vi "calibrateEvent.vi"(8 "error in (no error)":errorcluster, 11 "RampEvent in":refnum<class "RampEvent.lvclass">) -> (0 "error out":errorcluster, 3 "RampEvent out":refnum<class "RampEvent.lvclass">)   [LabVIEW 2011, in "Tools.lvlib" / "Scripting.lvlib" / "RampEvent.lvclass"]
uses:
  RampEvent.lvclass
  ScriptEvent.lvclass
  RampEvent.lvclass/RampEvent.ctl
  DatabaseHelpers/Database Objects/Channel/Channel.lvclass
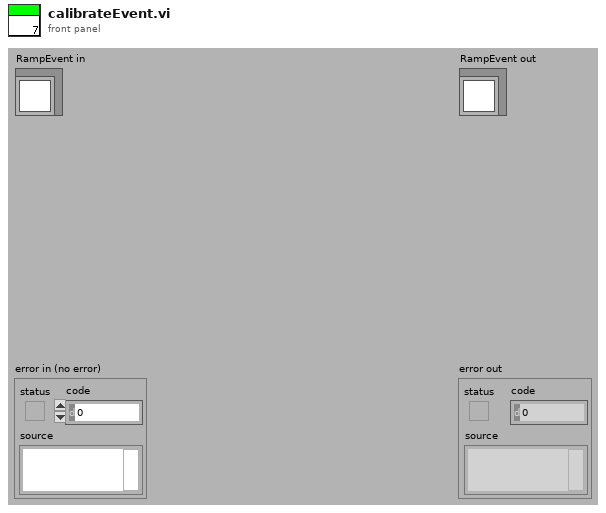
[diagram p1: front panel]
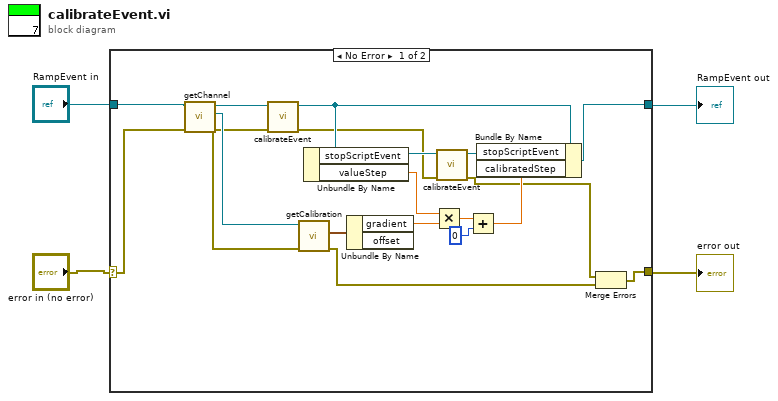
[diagram p0: block diagram]
diagram:
  n1 = case shown="No Error" "error in (no error)" {
    selector: "error in (no error)" -> [w14 w24]
    tunnel: [w10 w24] -> w4
    tunnel: [w22 w25] -> w3
    tunnel: "RampEvent in" -> [w15 w25]
    frame No Error {
      n2 = call-dynamic "getChannel.vi"("error in (no error)"=w14, "ScriptEvent.lvclass in"=w15) -> ("error out"=w12:errorcluster, "Channel.lvclass"=w13:refnum<class "Channel.lvclass">, "ScriptEvent.lvclass out"=w16:refnum<class "RampEvent.lvclass">)  [unwired: 7 in]
      n3 = call-parent "calibrateEvent.vi"("error in (no error)"=w12, "ScriptEvent in"=w16) -> ("error out"=w7:errorcluster, "ScriptEvent out"=w23:refnum<class "RampEvent.lvclass">)  [unwired: 8 in]
      n4 = call "getCalibration.vi"("error in (no error)"=w12, "Channel.lvclass in"=w13) -> ("error out"=w18:errorcluster, "calibration"=w21:cluster{"gradient":dbl, "offset":dbl})  [unwired: 7 in, 1 out]
      n5 = Unbundle By Name(w23) -> ("stopScriptEvent"=w8:refnum<class "ScriptEvent.lvclass">, "valueStep"=w17:dbl)
      n6 = Unbundle By Name(w21) -> ("gradient"=w20:dbl)  [unwired: 1 out]
      n7 = Multiply(x=w17, y=w20) -> (x*y=w19:dbl)
      n8 = call-dynamic "calibrateEvent.vi"("error in (no error)"=w7, "ScriptEvent in"=w8) -> ("error out"=w6:errorcluster, "ScriptEvent out"=w5:refnum<class "ScriptEvent.lvclass">)  [unwired: 8 in]
      n9 = Add(x=w19, y=0) -> (x+y=w11:dbl)
      n10 = Bundle By Name(cluster=w23, "stopScriptEvent"=w5, "calibratedStep"=w11) -> (w22:refnum<class "RampEvent.lvclass">)
      n11 = Merge Errors(w6, w18) -> (w10:errorcluster)
    }
    frame Error {
    }
  }
  "error out" <- w4
  "RampEvent out" <- w3
